vi "ExcecuteCommand.vi"(11 "Node":refnum<k20>) -> ()   [LabVIEW 2017]
uses:
  <resource>/objmgr/DOMUserDefRef.rc
panel:
  out "Node Name":string
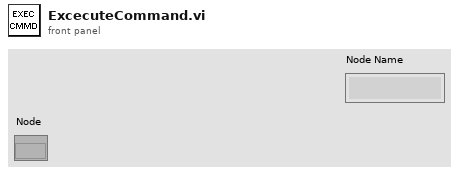
[diagram p1: front panel]
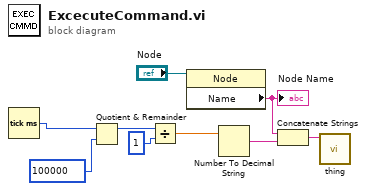
[diagram p0: block diagram]
diagram:
  n1 = Tick Count (ms)() -> (millisecond timer value=w1:u32)
  n2 = Quotient & Remainder(x=w1, y=u32 100000) -> (x-y*floor(x/y)=w5:u32)  [unwired: 1 out]
  n3 = Divide(x=w5, y=u32 1) -> (x/y=w3:dbl)
  n4 = property class="Node"(reference="Node") -> ("Name"=w8:string)  [unwired: 1 in, 2 out]
  "Node Name" <- w8
  n5 = Number To Decimal String(number=w3) -> (decimal integer string=w7:string)  [unwired: 1 in]
  n6 = Concatenate Strings(w8, w7) -> (w2:string)
  n7 = call "thing.vi"("String"=w2) -> ()  [unwired: 10 in, 1 out]
